vi "popen serial.vi"(5 "stop":i32, 6 "bits":i32, 7 "parity":i32, 9 "baudrate":i32, 10 "serdev":string, 11 "internal_buffering":i32) -> (2 "serdev out":string, 3 "resourceId":i32)   [LabVIEW 2010, in "libcommon_serial.lvlib"]
doc: "pserial_handle_t popen_serial(int internal_buffering,char*serdev,int baudrate,int parity,int bits,int stop);\npserial_handle_t popen_serial(int internal_buffering,const char*serdev,int baudrate,int parity,int bits,int stop);"
uses:
  <userlib>/libcommon_serial/libcommon_serial.lvlib
  <userlib>/libcommon_serial/libcommon_serial.so
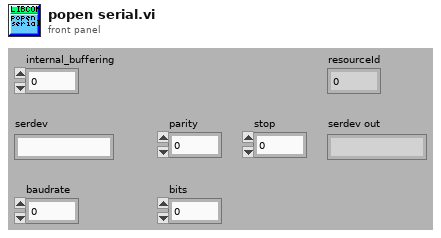
[diagram p1: front panel]
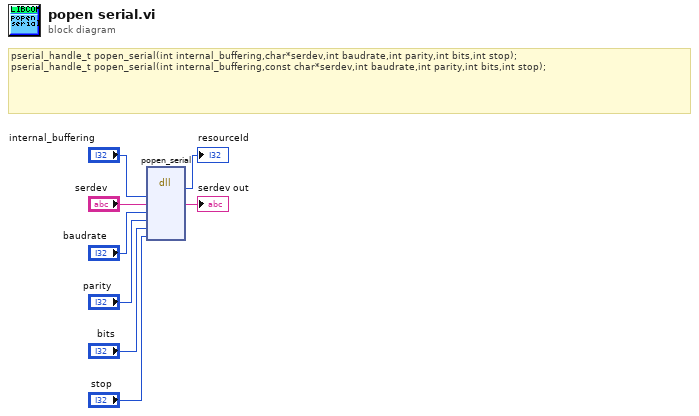
[diagram p0: block diagram]
diagram:
  # "pserial_handle_t popen_serial(int internal_buffering,char*serdev,int baudrate,int parity,int bits,int stop);\npserial_handle_t popen_serial(int internal_buffering,const char*serdev,int baudrate,int parity,int bits,int stop);"
  n1 = dll-call lib="usr/local/natinst/LabVIEW-2010/user.lib/libcommon_serial/libcommon_serial.*" fn="popen_serial"("internal_buffering"="internal_buffering", "serdev"="serdev", "baudrate"="baudrate", "parity"="parity", "bits"="bits", "stop"="stop") -> (→"resourceId":i32, "serdev"=→"serdev out":string)  [unwired: 8 in, 2 out]
